vi "WDT Get Waveform Time Array DBL.vi"(8 "error in (no error)":errorcluster, 11 "waveform in":waveform(dbl)) -> (0 "error out":errorcluster, 2 "X array":timestamp[](array[timestamp]))   [LabVIEW 2011]
doc: "Creates an array of waveform time stamps. Each element in the array is the time stamp for each data value in the waveform. Wire data to the <B>waveform in</B> input to determine the polymorphic instance to use or manually select the instance."
uses:
  <vilib>/Waveform/WDTOps.llb/WDT Number of Waveform Samples DBL.vi
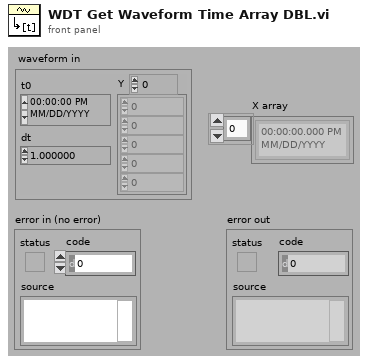
[diagram p1: front panel]
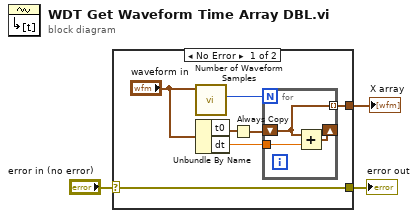
[diagram p0: block diagram]
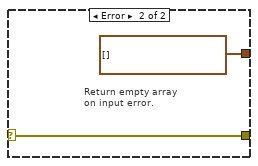
[diagram p2: hidden frame]
diagram:
  n1 = case shown="No Error" "error in (no error)" {
    selector: "error in (no error)" -> [w6 w15]
    tunnel: [w7 timestamp[] [] ("X array")] -> w3
    tunnel: [w6 w15] -> w2
    frame No Error {
      n2 = call-poly <vilib>:"Number of Waveform Samples.vi"("waveform in"="waveform in") -> ("number of samples"=w10:i32)  [unwired: 1 in, 9 out]
      n3 = Unbundle By Name("waveform in") -> ("t0"=w5:timestamp, "dt"=w8:dbl)
      n4 = Always Copy(1:w5) -> (0:w4:timestamp)
      n5 = for {
        N: w10 -> [_]
        shift-right: [w12] -> _
        shift-left: w4 -> [w11]
        tunnel: w8 -> [w13]
        tunnel: [w11] -> w7 mode=indexing
        n6 = Add(x=w11, y=w13) -> (x+y=w12:timestamp)
      }
    }
    frame Error {
      # "Return empty array\non input error."
    }
  }
  "error out" <- w2
  "X array" <- w3
